vi "test - Cluster Changed Value as Arguments.vi"(8 "error in (no error)":errorcluster, 11 "TestCase in":refnum<class "testcase-Supported-Datatype.lvclass">) -> (0 "error out":errorcluster, 3 "TestCase out":refnum<class "testcase-Supported-Datatype.lvclass">)   [LabVIEW 2017, in "testcase-Supported-Datatype.lvclass"]
uses:
  testcase-Supported-Datatype.lvclass
  53af2710-9492-4444-b21e-caf1361aab81.vi
  b1690b42-14fc-41e6-9711-d002cc3300e0.vi
  402ac8e1-063a-4cb4-aec8-123cda6c6106.vi
  75061575-983a-4300-85c5-60252db20c2a.vi
  addons/API-String-Arugments-Support/_Support/Data To API String Arguments.vi
  addons/API-String-Arugments-Support/_Support/Convert API String Arguments to Data(variant).vi
  <vilib>/addons/_JKI Toolkits/VI Tester/TestCase.llb/TestCase.lvclass
  C:/Program Files (x86)/National Instruments/LabVIEW 2017/vi.lib/addons/_JKI Toolkits/VI Tester/TestCase.llb/TestCase.lvclass
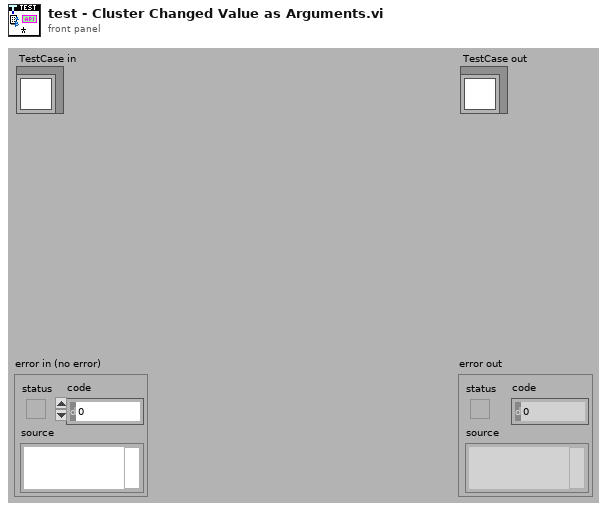
[diagram p1: front panel]
types:
  T1 = cluster{"Name":string, "Child":cluster{"Name":string}, "Bool":bool}
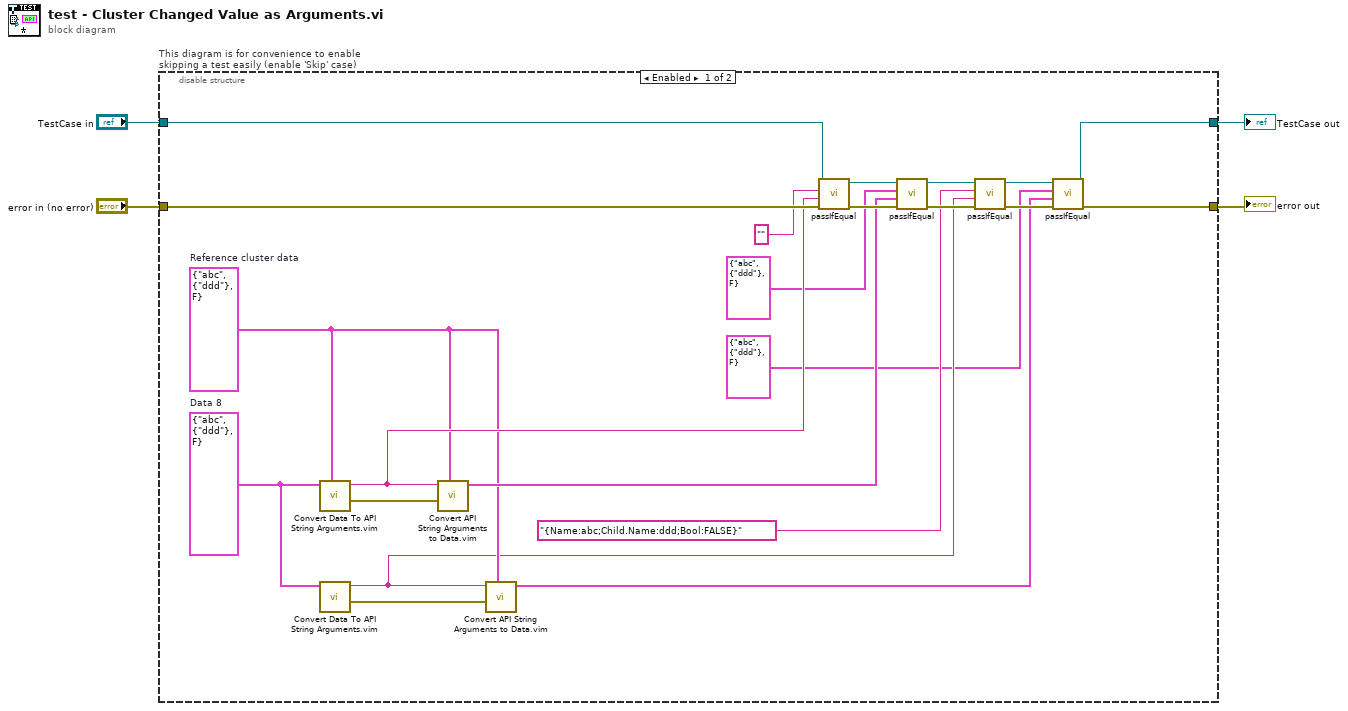
[diagram p0: block diagram]
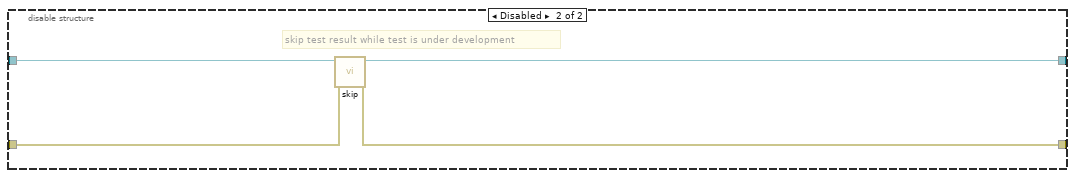
[diagram p2: hidden frame]
diagram:
  n1 = disable-structure "This diagram is for convenience to enable skipping a test easily (enable 'Skip' case)" shown="Enabled" {
    disable-tunnel: "TestCase in" -> [w25 w30]
    disable-tunnel: [w7 w28] -> w1
    disable-tunnel: [w8 w29] -> w3
    disable-tunnel: "error in (no error)" -> [w21 w27]
    frame Enabled {
      w14 = T1 {"Name"="abc", "Child"={"Name"="ddd"}, "Bool"=FALSE}  # Data 8
      w13 = T1 {"Name"="abc", "Child"={"Name"="ddd"}, "Bool"=FALSE}  # Reference cluster data
      n2 = call "Convert Data To API String Arguments.vim"("Reference Cluster Data"=w13, "Data"=w14) -> ("error out"=w20:errorcluster, "API String"=w19:string)  [unwired: 6 in]
      n3 = call "Convert Data To API String Arguments.vim"("Data"=w14) -> ("error out"=w15:errorcluster, "API String"=w11:string)  [unwired: 7 in]
      n4 = call "Convert API String Arguments to Data.vim"("Reference Type"=w13, "error in (no error)"=w20, "API String"=w19) -> ("Data"=w16:T1)  [unwired: 5 in, 1 out]
      n5 = call "Convert API String Arguments to Data.vim"("Reference Type"=w13, "error in (no error)"=w15, "API String"=w11) -> ("Data"=w6:T1)  [unwired: 5 in, 1 out]
      n6 = call-dynamic "passIfEqual.vi"("error in (no error)"=w21, "y"=w19, "x"="" ("String 16"), "TestCase in"=w25) -> ("error out"=w26:errorcluster, "TestCase out"=w24:refnum<class "testcase-Supported-Datatype.lvclass">)  [unwired: 6 in]
      n7 = call-dynamic "passIfEqual.vi"("error in (no error)"=w26, "y"=w16, "x"=T1 {"Name"="abc", "Child"={"Name"="ddd"}, "Bool"=FALSE} ("Data"), "TestCase in"=w24) -> ("error out"=w22:errorcluster, "TestCase out"=w23:refnum<class "testcase-Supported-Datatype.lvclass">)  [unwired: 6 in]
      n8 = call-dynamic "passIfEqual.vi"("error in (no error)"=w22, "y"=w11, "x"="{Name:abc;Child.Name:ddd;Bool:FALSE}" ("String 16"), "TestCase in"=w23) -> ("error out"=w10:errorcluster, "TestCase out"=w9:refnum<class "testcase-Supported-Datatype.lvclass">)  [unwired: 6 in]
      n9 = call-dynamic "passIfEqual.vi"("error in (no error)"=w10, "y"=w6, "x"=T1 {"Name"="abc", "Child"={"Name"="ddd"}, "Bool"=FALSE} ("Data"), "TestCase in"=w9) -> ("error out"=w8:errorcluster, "TestCase out"=w7:refnum<class "testcase-Supported-Datatype.lvclass">)  [unwired: 6 in]
    }
    frame Disabled {
      # "skip test result while test is under development"
      n10 = call <vilib>:"skip.vi"("error in (no error)"=w27, "TestCase in"=w30) -> ("error out"=w29:errorcluster, "TestCase out"=w28:refnum<class "testcase-Supported-Datatype.lvclass">)  [unwired: 8 in]
    }
  }
  "error out" <- w3
  "TestCase out" <- w1
